vi "Read HttpResponseMessage.vi"(8 "error in (no error)":errorcluster, 11 "HttpDownloadTask in":refnum<class "HttpDownloadTask.lvclass">) -> (0 "error out":errorcluster, 2 "LabVIEWHTTPClient_NET.lvlib:HttpResponseMessage.lvclass":refnum<class "HttpResponseMessage.lvclass">, 3 "HttpDownloadTask out":refnum<class "HttpDownloadTask.lvclass">)   [LabVIEW 2018, in "HttpClient_NET.lvlib" / "HttpDownloadTask.lvclass"]
uses:
  HttpDownloadTask.lvclass
  HttpResponseMessage/HttpResponseMessage.lvclass
  HttpDownloadTask.lvclass/HttpDownloadTask.ctl
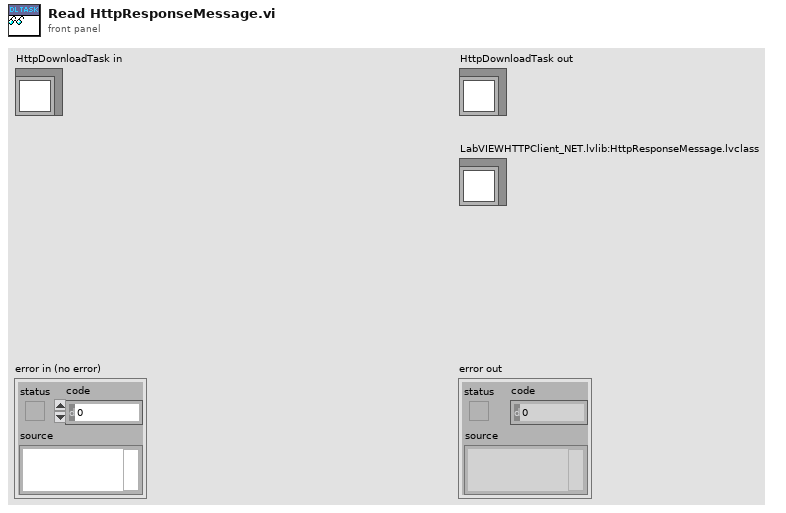
[diagram p1: front panel]
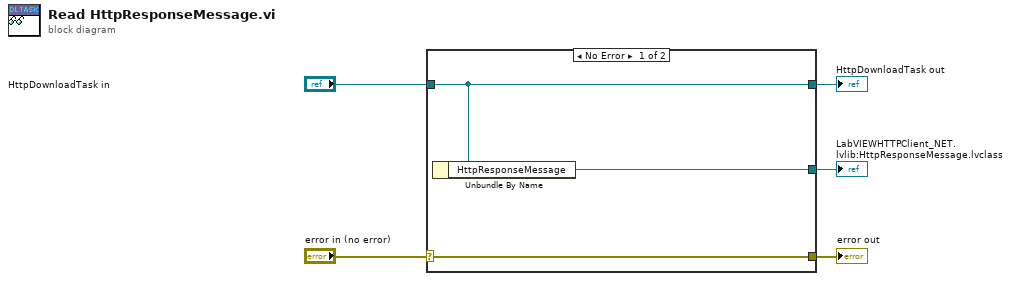
[diagram p0: block diagram]
diagram:
  n1 = case shown="No Error" "error in (no error)" {
    selector: "error in (no error)" -> [w8 w9]
    tunnel: [w8 w9] -> w4
    tunnel: [w7 w10] -> w2
    tunnel: "HttpDownloadTask in" -> [w7 w10]
    tunnel: [w6 _] -> w1
    frame No Error {
      n2 = Unbundle By Name(w7) -> ("HttpResponseMessage"=w6:refnum<class "HttpResponseMessage.lvclass">)
    }
    frame Error {
    }
  }
  "error out" <- w4
  "HttpDownloadTask out" <- w2
  "LabVIEWHTTPClient_NET.lvlib:HttpResponseMessage.lvclass" <- w1
